vi "Manual Test.vi"() -> ()   [LabVIEW 2020, in "driver_flodx_ph_probe.lvlib"]
doc: "Manually test all functions and commands of device"
uses:
  <instrlib>/RxnRover/FloDx Ph Probe Driver/driver_flodx_ph_probe.lvlib
panel:
  in  "Restart":bool
  in  "Set Address":sgl
  out "Address":dbl
  in  "Print Address":bool
  in  "Set Address":bool
  out "mid pH":dbl
  out "high pH":dbl
  out "Value":dbl
  out "SetTemp":dbl
  out "low pH":dbl
  out "Raw Response":string
  in  "Print High Calibration":bool
  in  "Print Low Calibration":bool
  in  "Print Mid Calibration":bool
  in  "Clear Configuration":bool
  in  "Print Compensation Temp":bool
  in  "Print ph":bool
  in  "Set Mid Calibration Ph":bool
  in  "Set Low Calibration Ph":bool
  in  "Exit Config":bool
  in  "Set Compensation Temp":bool
  in  "(1)Save (0)Reverts":sgl
  out "(1)Saved (0)Reverted":dbl
  out "pH":dbl
  out "Temp":dbl
  in  "Temperature":sgl
  in  "Calibration pH 3":sgl
  out "Deviation 2":dbl
  in  "Calibration pH 2":sgl
  out "mV measured":dbl
  in  "Enter CONFIG State":bool
  in  "Print Device Type":bool
  in  "Set High Calibration Ph":bool
  out "Deviation":dbl
  in  "Calibration pH":sgl
  out "ConfigState":bool
  out "Device Type":dbl
  in  "Address":u8
  in  "error in":errorcluster
  in  "VISA resource name":refnum<visa-resource-name>
  out "error out":errorcluster
  out "VISA resource name out":refnum<visa-resource-name>
  in  "Close Communication with Device":bool
  in  "Initialize  For Test DO THIS BEFORE RUNNING ANY TESTS":bool
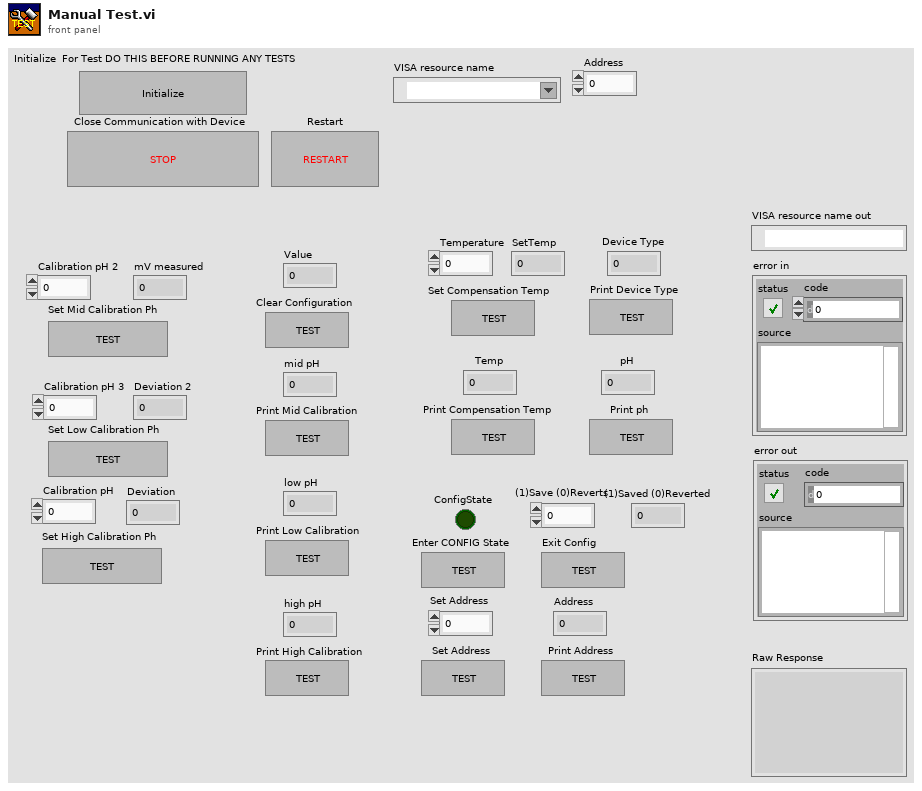
[diagram p1: front panel]
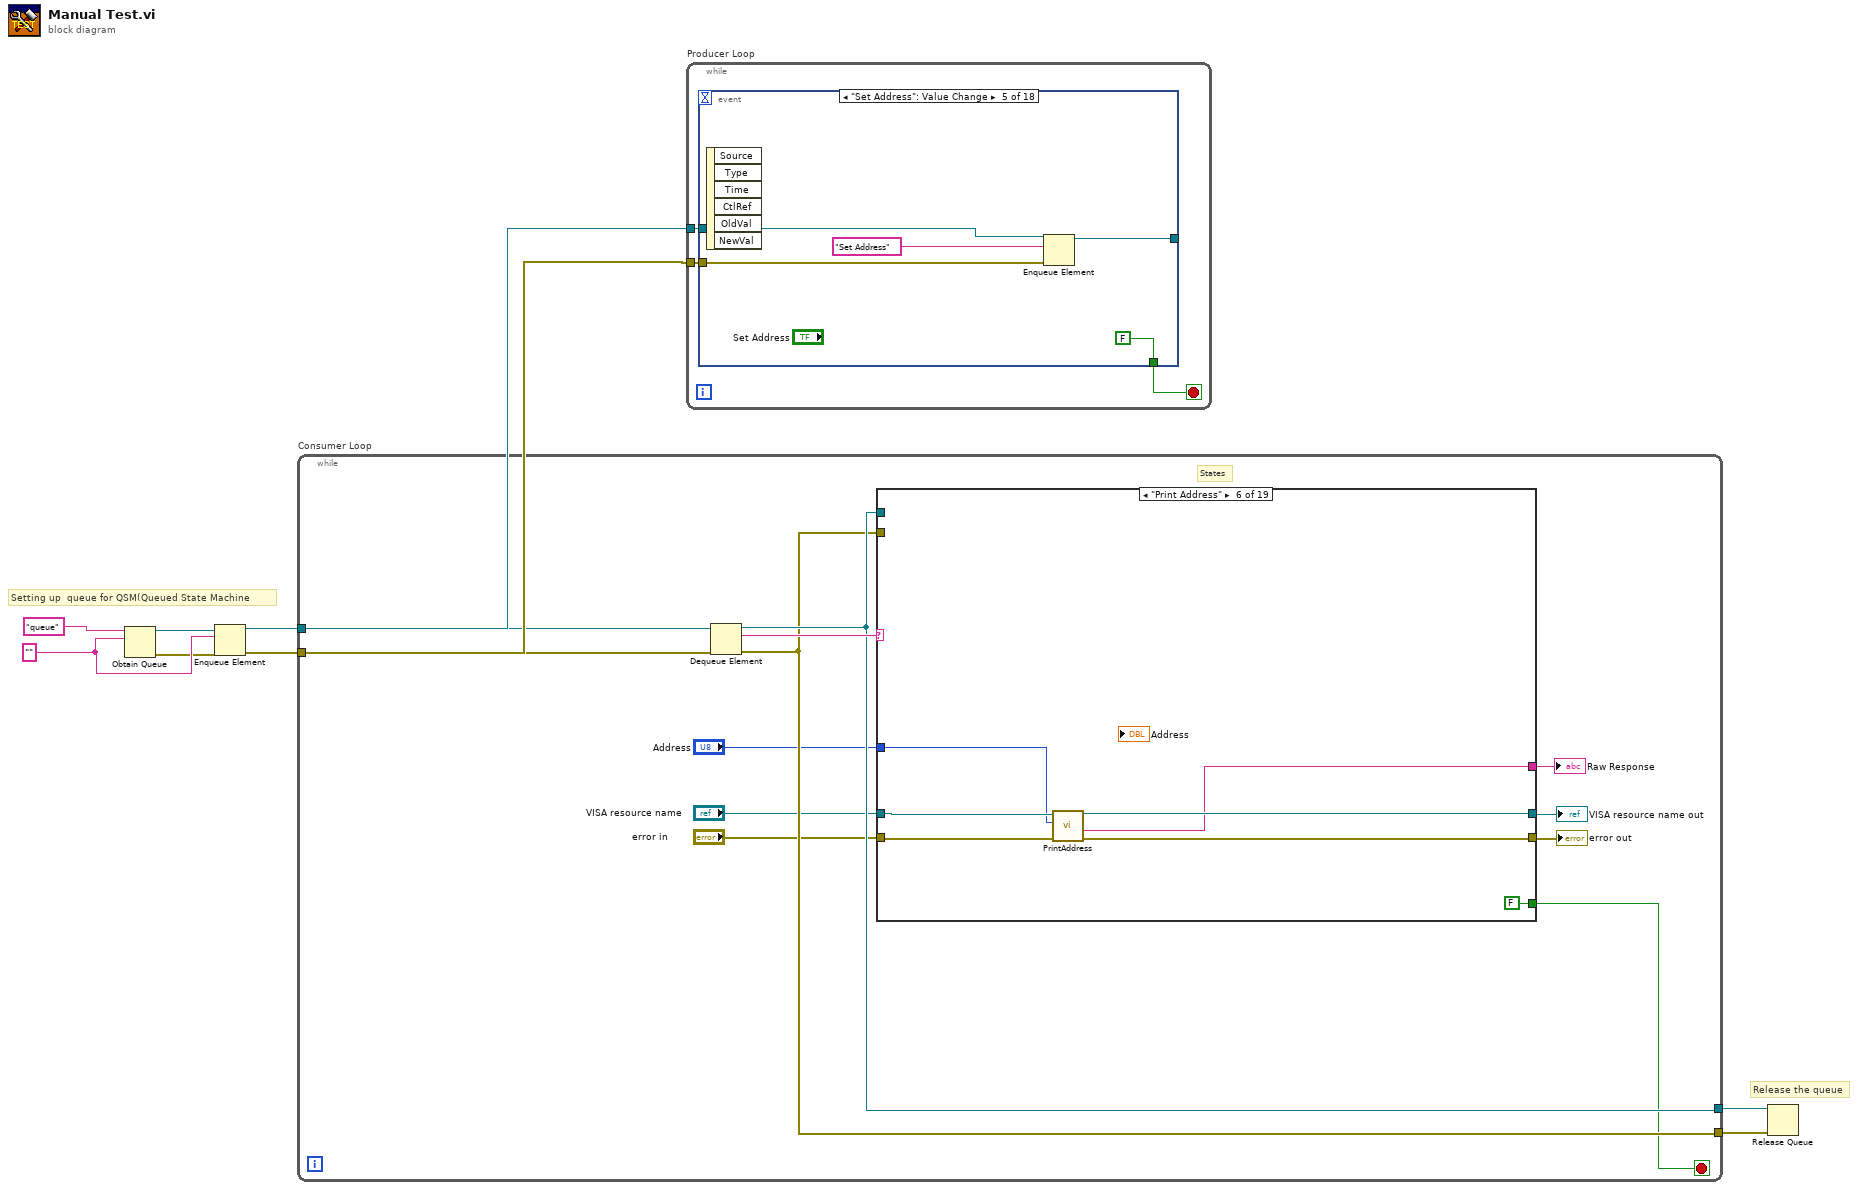
[diagram p0: block diagram]
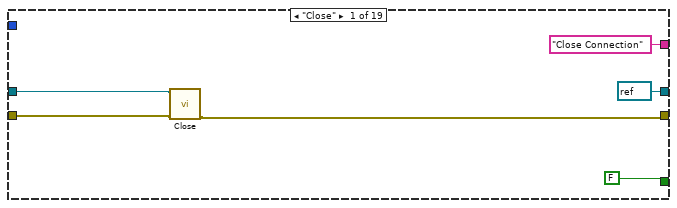
[diagram p2: hidden frame]
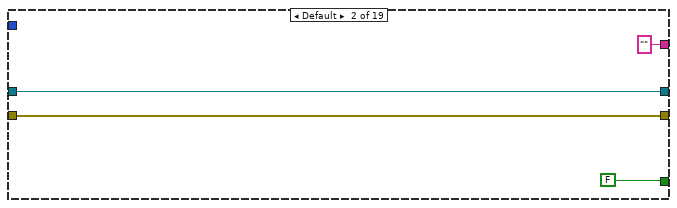
[diagram p3: hidden frame]
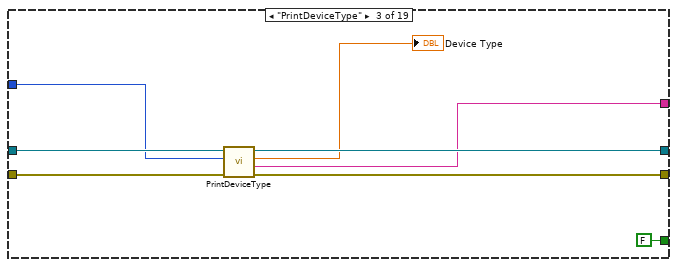
[diagram p4: hidden frame]
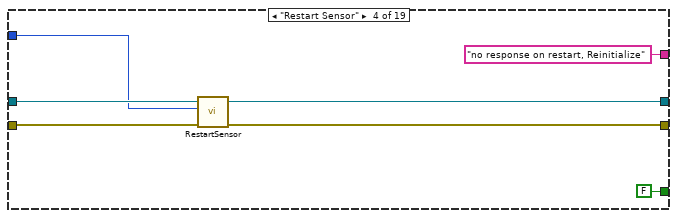
[diagram p5: hidden frame]
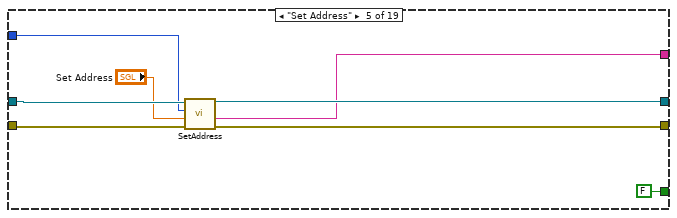
[diagram p6: hidden frame]
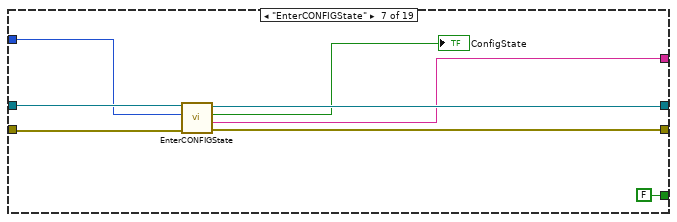
[diagram p7: hidden frame]
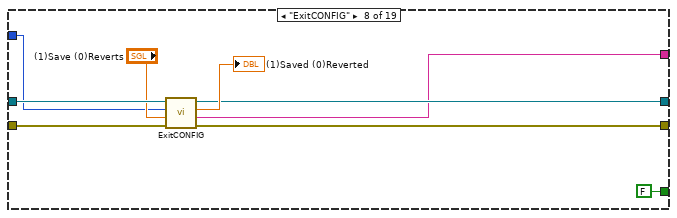
[diagram p8: hidden frame]
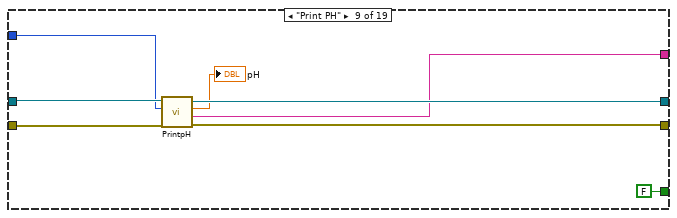
[diagram p9: hidden frame]
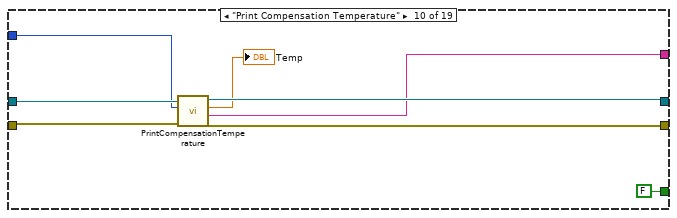
[diagram p10: hidden frame]
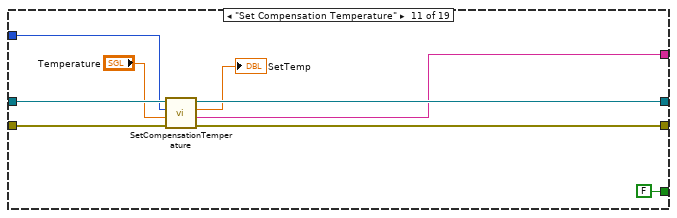
[diagram p11: hidden frame]
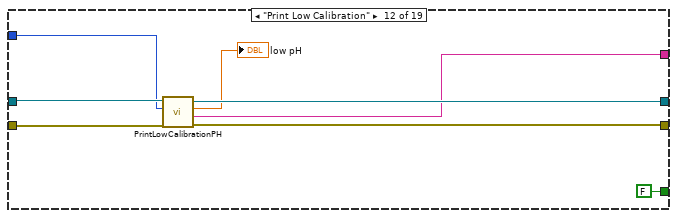
[diagram p12: hidden frame]
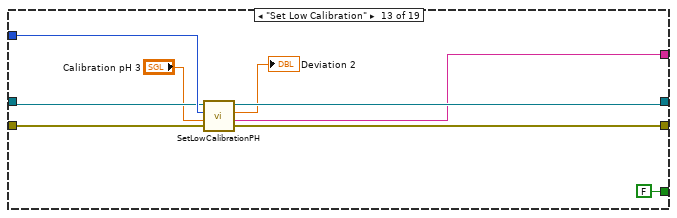
[diagram p13: hidden frame]
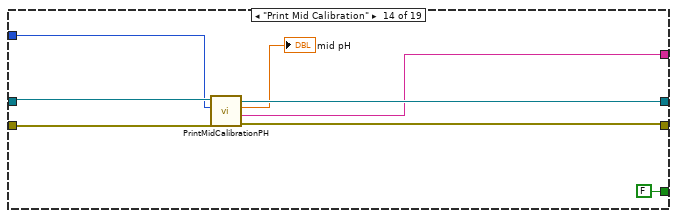
[diagram p14: hidden frame]
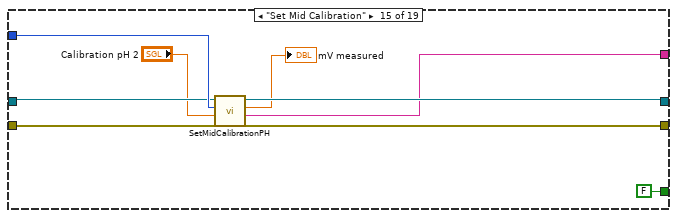
[diagram p15: hidden frame]
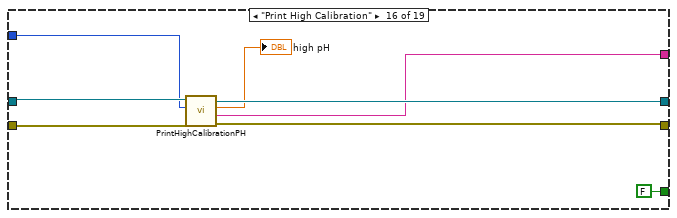
[diagram p16: hidden frame]
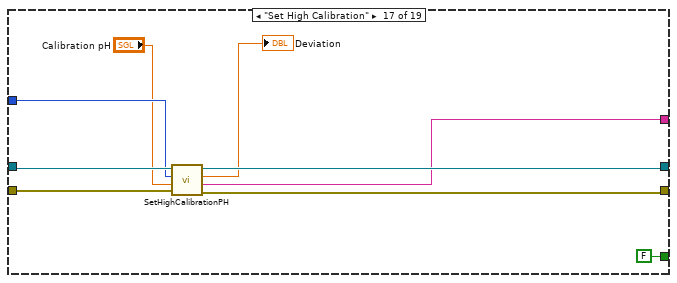
[diagram p17: hidden frame]
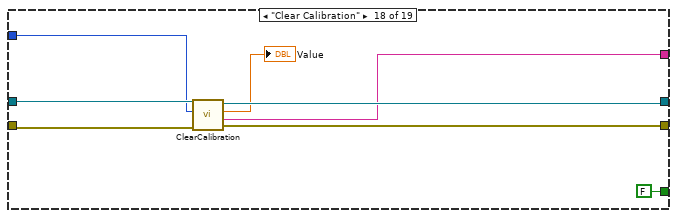
[diagram p18: hidden frame]
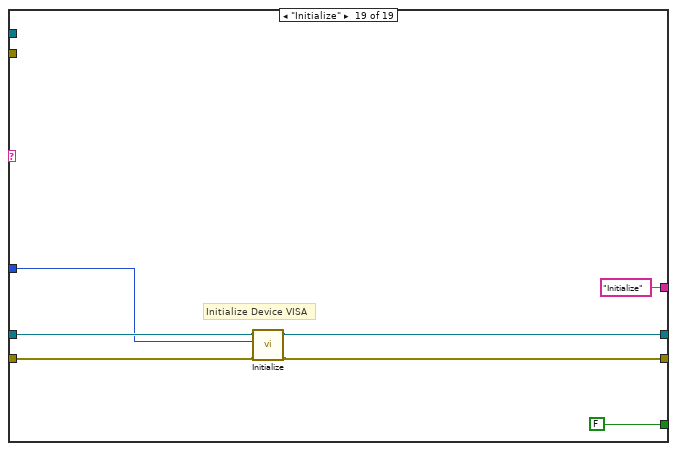
[diagram p19: hidden frame]
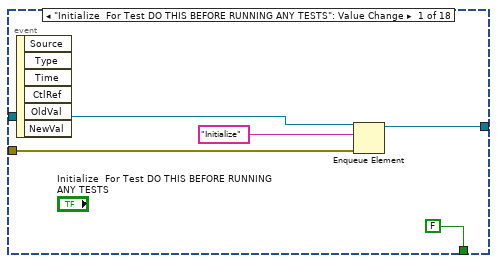
[diagram p20: hidden frame]
diagram:
  w7 = ""
  # "Release the queue"
  # "Setting up  queue for QSM(Queued State Machine"
  n1 = Obtain Queue(name (unnamed)="queue", element data type=w7) -> (queue out=w6:refnum<queue>, error out=w5:errorcluster)  [unwired: 3 in, 1 out]
  n2 = Enqueue Element(queue=w6, element=w7, error in (no error)=w5) -> (queue out=w1:refnum<queue>, error out=w2:errorcluster)  [unwired: 1 in, 1 out]
  n3 = while "Consumer Loop" {
    tunnel: [w17] -> w4
    tunnel: [w16] -> w3
    tunnel: w2 -> [w20]
    tunnel: w1 -> [w19]
    stop <- w11 stop-if-true
    # "States"
    n4 = Dequeue Element(queue=w19, error in (no error)=w20) -> (queue out=w17:refnum<queue>, element=w18:string, error out=w16:errorcluster)  [unwired: 1 in, 1 out]
    n5 = case shown="\"Print Address\"" w18 {
      tunnel: w17 -> [_ _ _ _ _ _ _ _ _ _ _ _ _ _ _ _ _ _ _]
      tunnel: w16 -> [_ _ _ _ _ _ _ _ _ _ _ _ _ _ _ _ _ _ _]
      tunnel: "VISA resource name" -> [w22 w30 w35 w45 w53 w60 w65 w74 w82 w89 w99 w107 w115 w124 w132 w141 w151 w158 w167]
      tunnel: "error in" -> [w23 w29 w34 w44 w46 w54 w66 w73 w81 w90 w100 w106 w114 w123 w131 w140 w150 w159 w164]
      tunnel: [refnum<visa-resource-name> refnum ("VISA resource name out") w30 w37 w41 w51 w58 w68 w75 w84 w93 w101 w108 w119 w125 w136 w142 w152 w161 w166] -> w13
      tunnel: [w24 w29 w38 w42 w52 w59 w67 w76 w85 w92 w102 w109 w118 w126 w135 w143 w153 w160 w165] -> w12
      tunnel: [FALSE FALSE FALSE FALSE FALSE FALSE FALSE FALSE FALSE FALSE FALSE FALSE FALSE FALSE FALSE FALSE FALSE FALSE FALSE] -> w11
      tunnel: "Address" -> [_ _ w33 w43 w47 w55 w64 w71 w80 w88 w98 w105 w116 w122 w133 w139 w149 w157 w162]
      tunnel: ["Close Connection" ("Raw Response") "" ("Raw Response") w31 "no response on restart, Reinitialize" ("Raw Response") w49 w56 w61 w69 w78 w86 w94 w103 w111 w120 w128 w137 w145 w154 "Initialize" ("Raw Response")] -> w10
      frame "Close" {
        n6 = call <instrlib>:"Close.vi"("error in (no error)"=w23, "VISA resource name"=w22) -> ("error out"=w24:errorcluster)  [unwired: 9 in]
      }
      frame Default {
      }
      frame "PrintDeviceType" {
        n7 = call <instrlib>:"PrintDeviceType.vi"("error in (no error)"=w34, "Address"=w33, "VISA resource name"=w35) -> ("error out"=w38:errorcluster, "Raw Response"=w31:string, "Device Type"=→"Device Type":dbl, "VISA resource name out"=w37:refnum<visa-resource-name>)  [unwired: 5 in]
      }
      frame "Restart Sensor" {
        n8 = call <instrlib>:"RestartSensor.vi"("error in (no error)"=w44, "Address"=w43, "VISA resource name"=w45) -> ("error out"=w42:errorcluster, "VISA resource name out"=w41:refnum<visa-resource-name>)  [unwired: 7 in]
      }
      frame "Set Address" {
        n9 = call <instrlib>:"SetAddress.vi"("error in (no error)"=w46, "Address(New)"="Set Address", "Address(Current)"=w47, "VISA resource name"=w53) -> ("error out"=w52:errorcluster, "Raw Response"=w49:string, "VISA resource name out"=w51:refnum<visa-resource-name>)  [unwired: 5 in]
      }
      frame "Print Address" {
        n10 = call <instrlib>:"PrintAddress.vi"("error in (no error)"=w54, "Address"=w55, "VISA resource name"=w60) -> ("error out"=w59:errorcluster, "Raw Response"=w56:string, "VISA resource name out"=w58:refnum<visa-resource-name>)  [unwired: 6 in]
      }
      frame "EnterCONFIGState" {
        n11 = call <instrlib>:"EnterCONFIGState.vi"("error in (no error)"=w66, "Address"=w64, "VISA resource name"=w65) -> ("error out"=w67:errorcluster, "Raw Response"=w61:string, "ConfigState"=→"ConfigState":bool, "VISA resource name out"=w68:refnum<visa-resource-name>)  [unwired: 5 in]
      }
      frame "ExitCONFIG" {
        n12 = call <instrlib>:"ExitCONFIG.vi"("error in (no error)"=w73, "(1)Save (0)Reverts"="(1)Save (0)Reverts", "Address"=w71, "VISA resource name"=w74) -> ("error out"=w76:errorcluster, "Raw Response"=w69:string, "(1)Saved (0)Reverted"=→"(1)Saved (0)Reverted":dbl, "VISA resource name out"=w75:refnum<visa-resource-name>)  [unwired: 4 in]
      }
      frame "Print PH" {
        n13 = call <instrlib>:"PrintpH.vi"("error in (no error)"=w81, "Address"=w80, "VISA resource name"=w82) -> ("error out"=w85:errorcluster, "Raw Response"=w78:string, "pH"=→"pH":dbl, "VISA resource name out"=w84:refnum<visa-resource-name>)  [unwired: 5 in]
      }
      frame "Print Compensation Temperature" {
        n14 = call <instrlib>:"PrintCompensationTemperature.vi"("error in (no error)"=w90, "Address"=w88, "VISA resource name"=w89) -> ("error out"=w92:errorcluster, "Raw Response"=w86:string, "Temp"=→"Temp":dbl, "VISA resource name out"=w93:refnum<visa-resource-name>)  [unwired: 5 in]
      }
      frame "Set Compensation Temperature" {
        n15 = call <instrlib>:"SetCompensationTemperature.vi"("error in"=w100, "Temperature"="Temperature", "Address"=w98, "VISA resource name"=w99) -> ("error out"=w102:errorcluster, "Raw Response"=w94:string, "SetTemp"=→"SetTemp":dbl, "VISA resource name out"=w101:refnum<visa-resource-name>)  [unwired: 4 in]
      }
      frame "Print Low Calibration" {
        n16 = call <instrlib>:"PrintLowCalibrationPH.vi"("error in (no error)"=w106, "Address"=w105, "VISA resource name"=w107) -> ("error out"=w109:errorcluster, "Raw Response"=w103:string, "low pH"=→"low pH":dbl, "VISA resource name out"=w108:refnum<visa-resource-name>)  [unwired: 5 in]
      }
      frame "Set Low Calibration" {
        n17 = call <instrlib>:"SetLowCalibrationPH.vi"("error in"=w114, "Calibration pH"="Calibration pH 3", "Address"=w116, "VISA resource name"=w115) -> ("error out"=w118:errorcluster, "Raw Response"=w111:string, "Deviation"=→"Deviation 2":dbl, "VISA resource name out"=w119:refnum<visa-resource-name>)  [unwired: 4 in]
      }
      frame "Print Mid Calibration" {
        n18 = call <instrlib>:"PrintMidCalibrationPH.vi"("error in (no error)"=w123, "Address"=w122, "VISA resource name"=w124) -> ("error out"=w126:errorcluster, "Raw Response"=w120:string, "mid pH"=→"mid pH":dbl, "VISA resource name out"=w125:refnum<visa-resource-name>)  [unwired: 5 in]
      }
      frame "Set Mid Calibration" {
        n19 = call <instrlib>:"SetMidCalibrationPH.vi"("error in"=w131, "Calibration pH"="Calibration pH 2", "Address"=w133, "VISA resource name"=w132) -> ("error out"=w135:errorcluster, "Raw Response"=w128:string, "mV measured"=→"mV measured":dbl, "VISA resource name out"=w136:refnum<visa-resource-name>)  [unwired: 4 in]
      }
      frame "Print High Calibration" {
        n20 = call <instrlib>:"PrintHighCalibrationPH.vi"("error in (no error)"=w140, "Address"=w139, "VISA resource name"=w141) -> ("error out"=w143:errorcluster, "Raw Response"=w137:string, "high pH"=→"high pH":dbl, "VISA resource name out"=w142:refnum<visa-resource-name>)  [unwired: 5 in]
      }
      frame "Set High Calibration" {
        n21 = call <instrlib>:"SetHighCalibrationPH.vi"("error in"=w150, "Calibration pH"="Calibration pH", "Address"=w149, "VISA resource name"=w151) -> ("error out"=w153:errorcluster, "Raw Response"=w145:string, "Deviation"=→"Deviation":dbl, "VISA resource name out"=w152:refnum<visa-resource-name>)  [unwired: 4 in]
      }
      frame "Clear Calibration" {
        n22 = call <instrlib>:"ClearCalibration.vi"("error in (no error)"=w159, "Address"=w157, "VISA resource name"=w158) -> ("error out"=w160:errorcluster, "Raw Response"=w154:string, "Value"=→"Value":dbl, "VISA resource name out"=w161:refnum<visa-resource-name>)  [unwired: 5 in]
      }
      frame "Initialize" {
        # "Initialize Device VISA"
        n23 = call <instrlib>:"Initialize.vi"("error in (no error)"=w164, "Address"=w162, "VISA resource name"=w167) -> ("error out"=w165:errorcluster, "VISA resource name out"=w166:refnum<visa-resource-name>)  [unwired: 6 in, 1 out]
      }
    }
    "error out" <- w12
    "VISA resource name out" <- w13
    "Raw Response" <- w10
  }
  n24 = while "Producer Loop" {
    tunnel: w2 -> [w171]
    tunnel: w1 -> [w170]
    stop <- w169 stop-if-true
    n25 = event shown="[4] \"Set Address\": Value Change" {
      selector: _ -> [_ _ _ _ _ _ _ _ _ _ _ _ _ _ _ _ _ _]
      dyn-events: _ -> [_ _ _ _ _ _ _ _ _ _ _ _ _ _ _ _ _ _]
      timeout: _ -> [_ _ _ _ _ _ _ _ _ _ _ _ _ _ _ _ _ _]
      tunnel: w171 -> [w175 w180 w185 w190 w195 w200 w205 w210 w215 w220 w225 w230 w235 w240 w245 w250 w255 w260]
      tunnel: w170 -> [w174 w179 w184 w189 w194 w199 w204 w209 w214 w219 w224 w229 w234 w239 w244 w249 w254 w259]
      tunnel: [w173 w178 w183 w188 w193 w198 w203 w208 w213 w218 w223 w228 w233 w238 w243 w248 w253 w258] -> _
      tunnel: [FALSE FALSE FALSE FALSE FALSE FALSE FALSE FALSE FALSE FALSE FALSE FALSE FALSE FALSE FALSE FALSE FALSE FALSE] -> w169
      event "Initialize  For Test DO THIS BEFORE RUNNING ANY TESTS": Value Change {
        n26 = event-data() -> ()  [unwired: 1 in, 6 out]
        n27 = Enqueue Element(queue=w174, element="Initialize", error in (no error)=w175) -> (queue out=w173:refnum<queue>)  [unwired: 1 in, 2 out]
      }
      event "Close Communication with Device": Value Change {
        n28 = event-data() -> ()  [unwired: 1 in, 6 out]
        n29 = Enqueue Element(queue=w179, element="Close", error in (no error)=w180) -> (queue out=w178:refnum<queue>)  [unwired: 1 in, 2 out]
      }
      event "Restart": Value Change {
        n30 = event-data() -> ()  [unwired: 1 in, 6 out]
        n31 = Enqueue Element(queue=w184, element="Restart Sensor", error in (no error)=w185) -> (queue out=w183:refnum<queue>)  [unwired: 1 in, 2 out]
      }
      event "Print Address": Value Change {
        n32 = event-data() -> ()  [unwired: 1 in, 6 out]
        n33 = Enqueue Element(queue=w189, element="Print Address", error in (no error)=w190) -> (queue out=w188:refnum<queue>)  [unwired: 1 in, 2 out]
      }
      event "Set Address": Value Change {
        n34 = event-data() -> ()  [unwired: 1 in, 6 out]
        n35 = Enqueue Element(queue=w194, element="Set Address", error in (no error)=w195) -> (queue out=w193:refnum<queue>)  [unwired: 1 in, 2 out]
      }
      event "Print High Calibration": Value Change {
        n36 = event-data() -> ()  [unwired: 1 in, 6 out]
        n37 = Enqueue Element(queue=w199, element="Print High Calibration", error in (no error)=w200) -> (queue out=w198:refnum<queue>)  [unwired: 1 in, 2 out]
      }
      event "Print Low Calibration": Value Change {
        n38 = event-data() -> ()  [unwired: 1 in, 6 out]
        n39 = Enqueue Element(queue=w204, element="Print Low Calibration", error in (no error)=w205) -> (queue out=w203:refnum<queue>)  [unwired: 1 in, 2 out]
      }
      event "Print Mid Calibration": Value Change {
        n40 = event-data() -> ()  [unwired: 1 in, 6 out]
        n41 = Enqueue Element(queue=w209, element="Print Mid Calibration", error in (no error)=w210) -> (queue out=w208:refnum<queue>)  [unwired: 1 in, 2 out]
      }
      event "Set Mid Calibration Ph": Value Change {
        n42 = event-data() -> ()  [unwired: 1 in, 6 out]
        n43 = Enqueue Element(queue=w214, element="Set Mid Calibration", error in (no error)=w215) -> (queue out=w213:refnum<queue>)  [unwired: 1 in, 2 out]
      }
      event "Set Low Calibration Ph": Value Change {
        n44 = event-data() -> ()  [unwired: 1 in, 6 out]
        n45 = Enqueue Element(queue=w219, element="Set Low Calibration", error in (no error)=w220) -> (queue out=w218:refnum<queue>)  [unwired: 1 in, 2 out]
      }
      event "Set High Calibration Ph": Value Change {
        n46 = event-data() -> ()  [unwired: 1 in, 6 out]
        n47 = Enqueue Element(queue=w224, element="Set High Calibration", error in (no error)=w225) -> (queue out=w223:refnum<queue>)  [unwired: 1 in, 2 out]
      }
      event "Clear Configuration": Value Change {
        n48 = event-data() -> ()  [unwired: 1 in, 6 out]
        n49 = Enqueue Element(queue=w229, element="Clear Calibration", error in (no error)=w230) -> (queue out=w228:refnum<queue>)  [unwired: 1 in, 2 out]
      }
      event "Print Compensation Temp": Value Change {
        n50 = event-data() -> ()  [unwired: 1 in, 6 out]
        n51 = Enqueue Element(queue=w234, element="Print Compensation Temperature", error in (no error)=w235) -> (queue out=w233:refnum<queue>)  [unwired: 1 in, 2 out]
      }
      event "Print ph": Value Change {
        n52 = event-data() -> ()  [unwired: 1 in, 6 out]
        n53 = Enqueue Element(queue=w239, element="Print PH", error in (no error)=w240) -> (queue out=w238:refnum<queue>)  [unwired: 1 in, 2 out]
      }
      event "Exit Config": Value Change {
        n54 = event-data() -> ()  [unwired: 1 in, 6 out]
        n55 = Enqueue Element(queue=w244, element="ExitCONFIG", error in (no error)=w245) -> (queue out=w243:refnum<queue>)  [unwired: 1 in, 2 out]
      }
      event "Set Compensation Temp": Value Change {
        n56 = event-data() -> ()  [unwired: 1 in, 6 out]
        n57 = Enqueue Element(queue=w249, element="Set Compensation Temperature", error in (no error)=w250) -> (queue out=w248:refnum<queue>)  [unwired: 1 in, 2 out]
      }
      event "Enter CONFIG State": Value Change {
        n58 = event-data() -> ()  [unwired: 1 in, 6 out]
        n59 = Enqueue Element(queue=w254, element="EnterCONFIGState", error in (no error)=w255) -> (queue out=w253:refnum<queue>)  [unwired: 1 in, 2 out]
      }
      event "Print Device Type": Value Change {
        n60 = event-data() -> ()  [unwired: 1 in, 6 out]
        n61 = Enqueue Element(queue=w259, element="PrintDeviceType", error in (no error)=w260) -> (queue out=w258:refnum<queue>)  [unwired: 1 in, 2 out]
      }
    }
  }
  n62 = Release Queue(queue=w4, error in (no error)=w3) -> ()  [unwired: 1 in, 3 out]
